vi "Interface.Get Response FIFO.vi"(11 "Interface in":refnum<class "Interface.lvclass">) -> (2 "Response FIFO":T1, 3 "Interface out":refnum<class "Interface.lvclass">)   [LabVIEW 2017, in "DSF.Engine.lvlib" / "Interface.lvclass"]
uses:
  Interface.lvclass
  Interface.RT FIFO.Ref.16B.ctl
  Interface.RT FIFO.Data.16B.ctl
  Interface.RT FIFO.Payload.16B.ctl
  Interface.lvclass/Interface.ctl
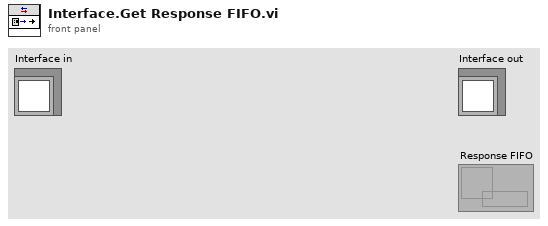
[diagram p1: front panel]
types:
  T1 = typedef "DSF.Engine.lvlib/Interface.lvclass/Interface.RT FIFO.Ref.16B.ctl" = refnum<k33>
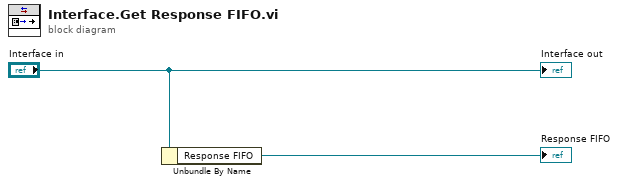
[diagram p0: block diagram]
diagram:
  n1 = Unbundle By Name("Interface in") -> ("Response FIFO"=→"Response FIFO":T1)
  "Interface out" <- "Interface in"
